vi "HVSConvertStatusStringToData.vi"(8 "error in (no error)":errorcluster, 10 "String":string, 11 "?":T1) -> (0 "error out":errorcluster, 3 "?":T1)   [LabVIEW 2013]
uses:
  HVSmeasurementCluster.ctl
panel:
  in  "String 2":string
  out "Valid Data":bool
  out "value":dbl[](array[numeric])
  # "Report Date Time, Barometric Pressure (mmHg), Ambient Temperature (°C)\n, Wind speed (m/s), Wind direction (°), Sigma Theta (standard deviation for wind direction), \nRainfall (bucket tips), Flow-rate (m3/h), Corrected accumulated sample volume (standard m3), \nUncorrected accumulated sample volume (m3)"
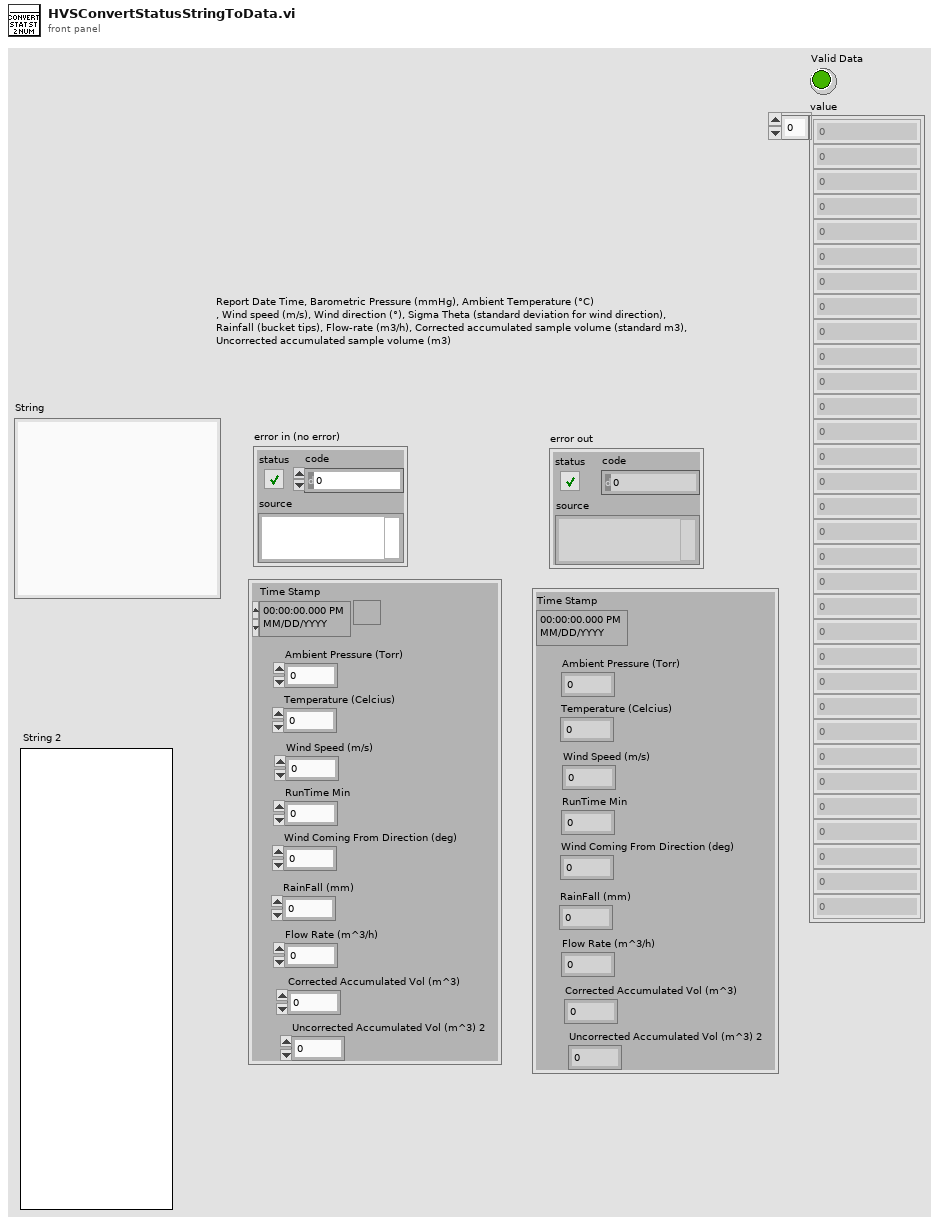
[diagram p1: front panel]
types:
  T1 = typedef "HVSmeasurementCluster.ctl" = cluster{"Time Stamp":timestamp, "Ambient Pressure (Torr)":dbl, "Temperature (Celcius)":dbl, "Wind Speed (m/s)":dbl, "RunTime Min":dbl, "Wind Coming From Direction (deg)":dbl, "RainFall (mm)":dbl, "Flow Rate (m^3/h)":dbl, "Corrected Accumulated Vol (m^3)":dbl, "Uncorrected Accumulated Vol (m^3) 2":dbl}
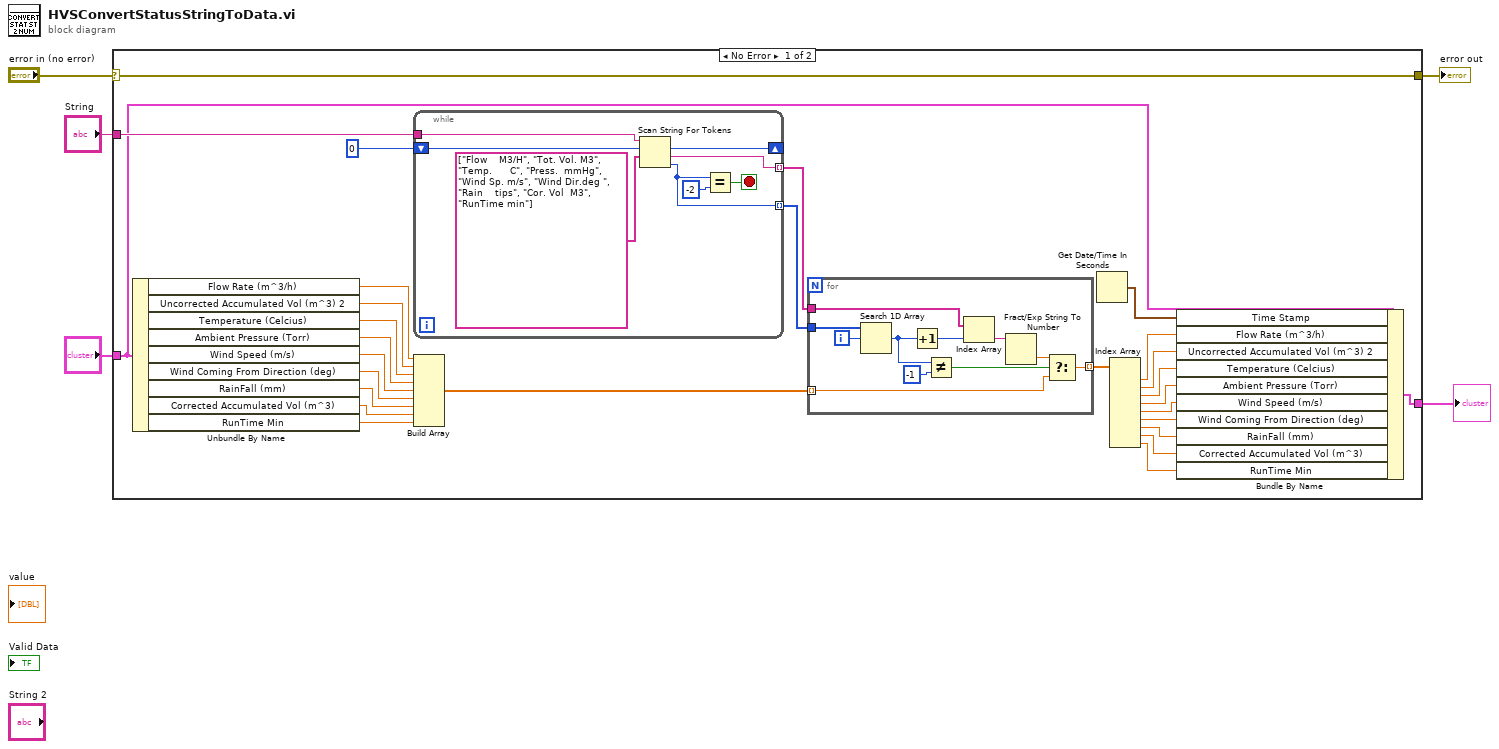
[diagram p0: block diagram]
diagram:
  n1 = case shown="No Error" "error in (no error)" {
    selector: "error in (no error)" -> [w33 w53]
    tunnel: "String" -> [w30 _]
    tunnel: [w33 w53] -> w3
    tunnel: "?" -> [w29 _]
    tunnel: [w7 _] -> w1
    frame No Error {
      n2 = Unbundle By Name(w29) -> ("Flow Rate (m^3/h)"=w28:dbl, "Uncorrected Accumulated Vol (m^3) 2"=w27:dbl, "Temperature (Celcius)"=w26:dbl, "Ambient Pressure (Torr)"=w25:dbl, "Wind Speed (m/s)"=w24:dbl, "Wind Coming From Direction (deg)"=w23:dbl, "RainFall (mm)"=w22:dbl, "Corrected Accumulated Vol (m^3)"=w21:dbl, "RunTime Min"=w20:dbl)
      n3 = while {
        tunnel: w30 -> [w51]
        shift-right: [w50] -> _
        shift-left: 0 ("offset past token") -> [w49]
        tunnel: [w48] -> w19 mode=indexing
        tunnel: [w45] -> w32 mode=indexing
        stop <- w46 stop-if-true
        n4 = Scan String For Tokens(7:string[] ["Flow    M3/H", "Tot. Vol. M3", "Temp.      C", "Press.  mmHg", "Wind Sp. m/s", "Wind Dir.deg ", "Rain    tips", "Cor. Vol  M3", "RunTime min"] ("operators (none)"), 8:w49, 9:w51) -> (0:w45:i32, 1:w48:string, 2:w50:i32)  [unwired: 3 in, 1 out]
        n5 = Equal?(x=w45, y=-2) -> (x = y?=w46:bool)
      }
      n6 = Build Array(w28, w27, w26, w25, w24, w23, w22, w21, w20) -> (w18:dbl[])
      n7 = for {
        tunnel: w19 -> [w42]
        tunnel: w32 -> [w41]
        tunnel: w18 -> [w35] mode=indexing
        tunnel: [w34] -> w17 mode=indexing
        i -> [w36]
        n8 = Search 1D Array(1D array=w41, element=w36) -> (index of element=w40:i32)  [unwired: 1 in]
        n9 = Increment(x=w40) -> (x+1=w44:i32)
        n10 = Not Equal?(x=w40, y=-1) -> (x != y?=w38:bool)
        n11 = Index Array(array=w42, index=w44) -> (element=w43:string)
        n12 = Fract/Exp String To Number(string=w43) -> (number=w37:dbl)  [unwired: 3 in, 1 out]
        n13 = Select(t=w37, s=w38, f=w35) -> (s? t:f=w34:dbl)
      }
      n14 = Get Date/Time In Seconds() -> (seconds since 1Jan1904=w6:timestamp)
      n15 = Index Array(array=w17) -> (element #1=w16:dbl, element #2=w15:dbl, element #3=w14:dbl, element #4=w13:dbl, element #5=w12:dbl, element #6=w11:dbl, element #7=w10:dbl, element #8=w9:dbl, element #9=w8:dbl)  [unwired: 9 in]
      n16 = Bundle By Name(cluster=w29, "Time Stamp"=w6, "Flow Rate (m^3/h)"=w16, "Uncorrected Accumulated Vol (m^3) 2"=w15, "Temperature (Celcius)"=w14, "Ambient Pressure (Torr)"=w13, "Wind Speed (m/s)"=w12, "Wind Coming From Direction (deg)"=w11, "RainFall (mm)"=w10, "Corrected Accumulated Vol (m^3)"=w9, "RunTime Min"=w8) -> (w7:T1)
    }
    frame Error {
    }
  }
  "error out" <- w3
  "?" <- w1
